vi "Add Oneof Indices To Metadata.vi"(11 "Messages MetaData":T1[](array[typedef])) -> (3 "Messages Metadata With Oneof Indices":T1[](array[typedef]))   [LabVIEW 2019, in "gRPC Template Creation Utility.lvlib"]
uses:
  gRPC Template Creation Utility.lvlib
  TypeDefs/Message Metadata (Scripting).ctl
  TypeDefs/Message Element Metadata (Scripting).ctl
  TypeDefs/Message Element Type.ctl
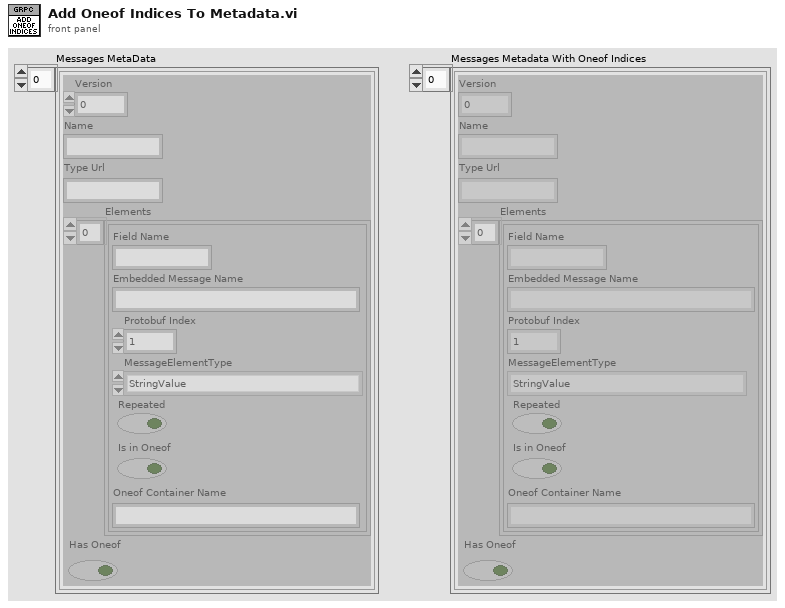
[diagram p1: front panel]
types:
  T1 = typedef "gRPC Template Creation Utility.lvlib/Message Metadata (Scripting).ctl" = cluster{"Version":i32, "Name":string, "Type Url":string, "Elements":T2[], "Has Oneof":bool}
  T2 = typedef "gRPC Template Creation Utility.lvlib/Message Element Metadata (Scripting).ctl" = cluster{"Field Name":string, "Embedded Message Name":string, "Protobuf Index":i32, "MessageElementType":T3, "Repeated":bool, "Is in Oneof":bool, "Oneof Container Name":string}
  T3 = typedef "gRPC Template Creation Utility.lvlib/Message Element Type.ctl" = enum32{"Int32Value", "FloatValue", "DoubleValue", "BoolValue", "StringValue", "MessageValue", "Int64Value", "UInt32Value", "UInt64Value", "EnumValue", "Bytes", "Fixed64", "Fixed32", "SFixed64", "SFixed32", "SInt64", "SInt32"}
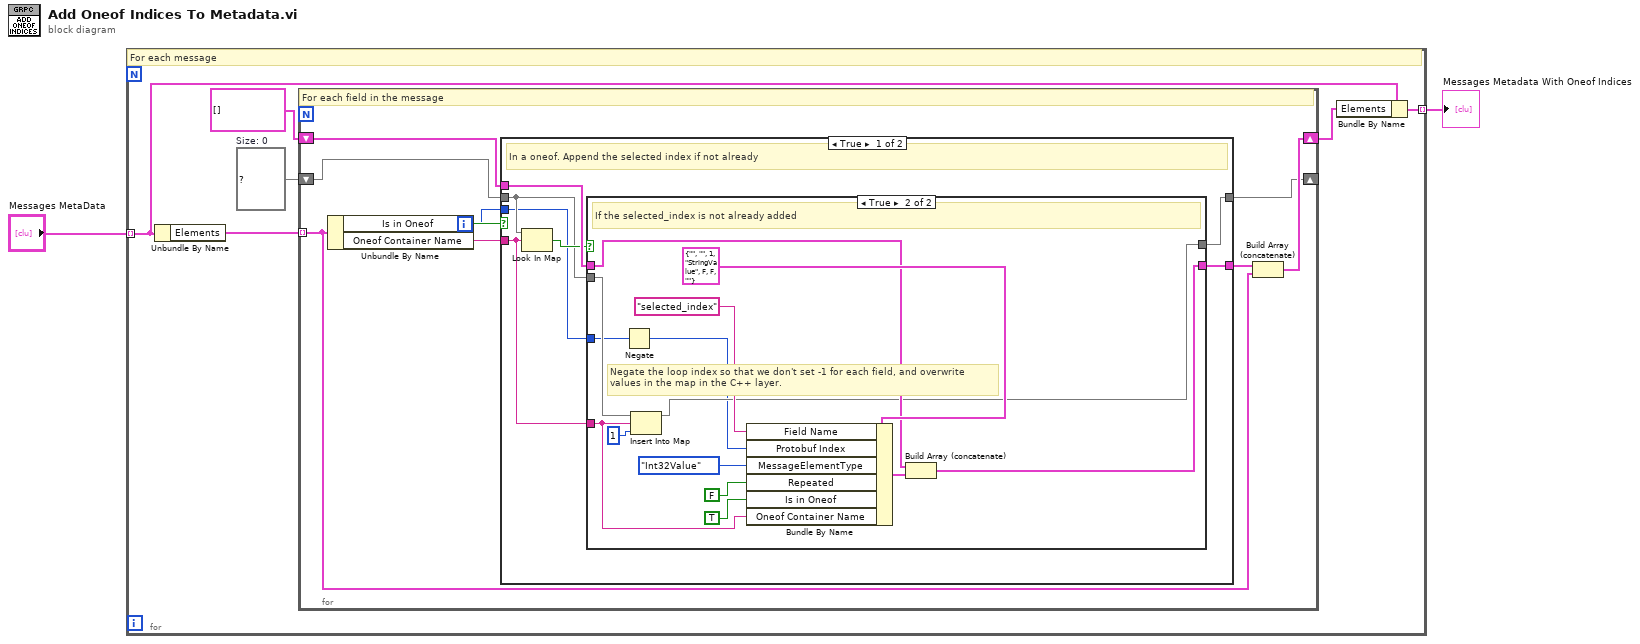
[diagram p0: block diagram]
diagram:
  n1 = for {
    tunnel: "Messages MetaData" -> [w4] mode=indexing
    tunnel: [w3] -> w2 mode=indexing
    w7 = map{string, i32} {}  # Size: 0
    # "For each message"
    n2 = Unbundle By Name(w4) -> ("Elements"=w8:T2[])
    n3 = for {
      shift-right: [w12] -> w5
      shift-left: T2[] [] -> [w16]
      tunnel: w8 -> [w13] mode=indexing
      shift-right: [w10] -> _
      shift-left: w7 -> [w11]
      i -> [w9]
      # "For each field in the message"
      n4 = Unbundle By Name(w13) -> ("Is in Oneof"=w17:bool, "Oneof Container Name"=w15:string)
      n5 = case shown="True" w17 {
        tunnel: w16 -> [w24 w42]
        tunnel: w15 -> [w22 _]
        tunnel: [w23 w42] -> w14
        tunnel: w11 -> [w20 w41]
        tunnel: [w19 w41] -> w10
        tunnel: w9 -> [w18 _]
        frame True {
          # "In a oneof. Append the selected index if not already"
          n6 = Look In Map(map=w20, key=w22) -> (key not found?=w21:bool)  [unwired: 1 in, 1 out]
          n7 = case shown="True" w21 {
            tunnel: w22 -> [_ w31]
            tunnel: w24 -> [w26 w34]
            tunnel: [w26 w33] -> w23
            tunnel: w20 -> [w25 w32]
            tunnel: [w25 w29] -> w19
            tunnel: w18 -> [_ w28]
            frame False {
            }
            frame True {
              # "Negate the loop index so that we don't set -1 for each field, and overwrite\nvalues in the map in the C++ layer."
              # "If the selected_index is not already added"
              n8 = Negate(x=w28) -> (-x=w27:i32)
              n9 = Insert Into Map(map in=w32, key=w31, value=1) -> (map out=w29:map{string, i32})  [unwired: 2 out]
              n10 = Bundle By Name(cluster=T2 {"Field Name"="", "Embedded Message Name"="", "Protobuf Index"=1, "MessageElementType"=enum."StringValue", "Repeated"=FALSE, "Is in Oneof"=FALSE, "Oneof Container Name"=""} ("MessageElementMetadata"), "Field Name"="selected_index", "Protobuf Index"=w27, "MessageElementType"=Message_Element_Type."Int32Value", "Repeated"=FALSE, "Is in Oneof"=TRUE, "Oneof Container Name"=w31) -> (w35:T2)
              n11 = Build Array (concatenate)(w34, w35) -> (w33:T2[])
            }
          }
        }
        frame False {
          # "Not in a oneof. Just append to the metadata fields"
        }
      }
      n12 = Build Array (concatenate)(w14, w13) -> (w12:T2[])
    }
    n13 = Bundle By Name(cluster=w4, "Elements"=w5) -> (w3:T1)
  }
  "Messages Metadata With Oneof Indices" <- w2
